vi "Test Edit Palette List Dialog.vi"() -> ()   [LabVIEW 2021, in "Palette.lvlib"]
uses:
  Palette.lvlib
panel:
  out "Palette List (out)":string[](array[string])
  in  "Palette List (in)":string[](array[string])
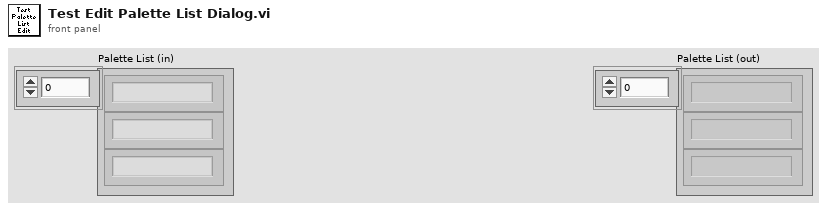
[diagram p1: front panel]
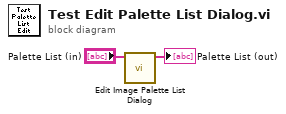
[diagram p0: block diagram]
diagram:
  n1 = call "Edit Image Palette List Dialog.vi"("Palette List (in)"="Palette List (in)") -> ("Palette List (out)"=→"Palette List (out)":string[])  [unwired: 10 in]
